vi "RSZVB Save Calibration Kit Ports.vi"(6 "VNA Ports":i32[](array[numeric]), 7 "Cal Unit Ports":i32[](array[numeric]), 8 "error in (no error)":errorcluster {"code" format="%.0x"}, 9 "Parameters (Full N-port)":i32(ring)=10 items=["Default"=0, "Full One Port"=2, "Full N-port"=10], 10 "File Name (\"\")":string, 11 "VISA resource name":refnum<visa-resource-name>) -> (0 "error out":errorcluster {"code" format="%.0x"}, 3 "VISA resource name out":refnum<visa-resource-name>)   [LabVIEW 2011]
doc: "This VI generates a cal kit file with the specified name containing the cal kit data of the active calibration unit. The cal kit file can be stored in the calibration unit or written to a directory on the analyzer. \n\nRemote-control command(s):\n[SENSe<Ch>:]CORRection:COLLect:AUTO:CKIT:PORTs"
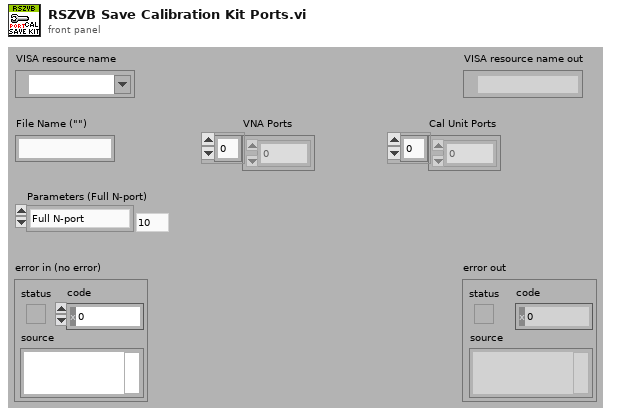
[diagram p1: front panel]
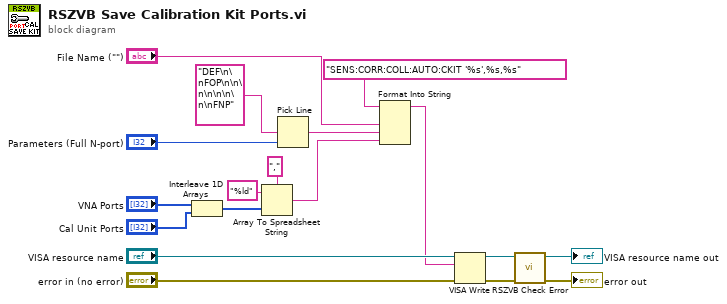
[diagram p0: block diagram]
diagram:
  n1 = Interleave 1D Arrays("VNA Ports", "Cal Unit Ports") -> (w7:i32[])
  n2 = Array To Spreadsheet String(delimiter (Tab)=",", array=w7, 3:"%ld" ("format string")) -> (spreadsheet string=w4:string)
  n3 = Pick Line(multi-line string="DEF\n\nFOP\n\n\n\n\n\n\n\nFNP", line index="Parameters (Full N-port)") -> (output string=w12:string)  [unwired: 1 in]
  n4 = Format Into String(format string="SENS:CORR:COLL:AUTO:CKIT '%s',%s,%s", "File Name (\"\")", w12, w4) -> (resulting string=w1:string)  [unwired: 2 in, 1 out]
  n5 = VISA Write(VISA resource name="VISA resource name", write buffer=w1, error in (no error)="error in (no error)") -> (VISA resource name out=w17:refnum<visa-resource-name>, error out=w16:errorcluster)  [unwired: 1 out]
  n6 = call "RSZVB Check Error.vi"("error in (no error)"=w16, "VISA session"=w17) -> ("error out"=→"error out":errorcluster, "dup VISA session"=→"VISA resource name out":refnum<visa-resource-name>)  [unwired: 8 in]
